vi "Send Latest File.vi"(4 "Attachment Settings":T1={"Attachment Size"=1.0, "Resize Type"=enum."Size"} {"Attachment Size" scale=0.0..1.0 scale format="%#_2f"}, 5 "Contact":T2, 6 "Most Recently Modified Image Path":path, 7 "Action on Error":T3(ring), 8 "error in":errorcluster, 9 "Email Password":string="apatite2Z", 10 "Email Username":string="raymond.apatite@gmail.com", 11 "SMTP Server":string="smtp.gmail.com") -> (0 "error out":errorcluster)   [LabVIEW 2013]
uses:
  <vilib>/vision/NI_Vision_Development_Module.lvlib
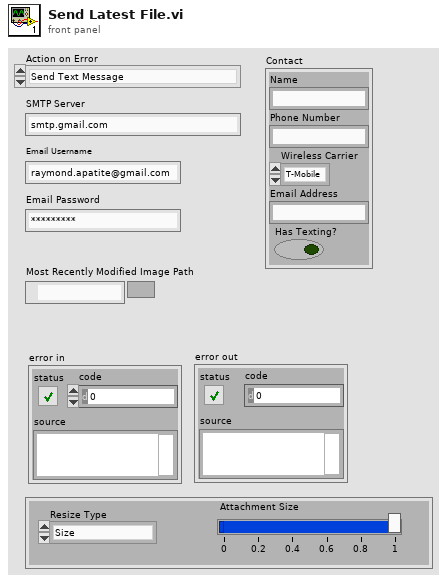
[diagram p1: front panel]
types:
  T1 = cluster{"Attachment Size":dbl, "Resize Type":enum16{"Size", "Resolution"}}
  T2 = cluster{"Name":string, "Phone Number":string, "Wireless Carrier":enum16{"T-Mobile", "AT&T", "Verizon", "Sprint"}, "Email Address":string, "Has Texting?":bool}
  T3 = enum16{"Send Text Message", "Send Email", "Send Text Message & Email"}
  T4 = typedef "Image Type" = u32
  T5 = typedef "IMAQ Image.ctl" = refnum<image>
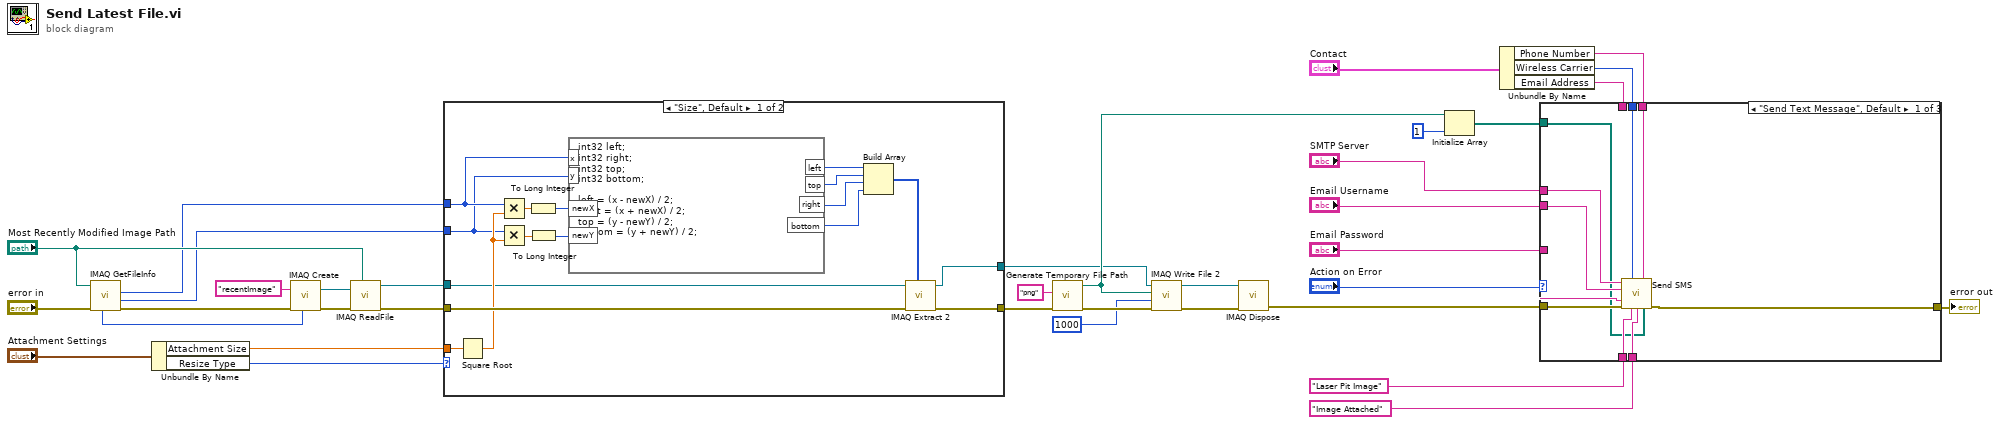
[diagram p0: block diagram]
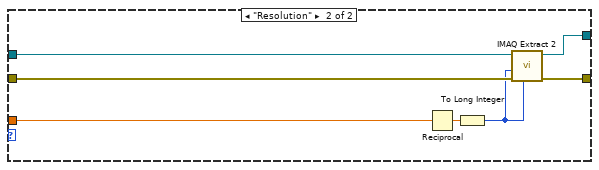
[diagram p2: hidden frame]
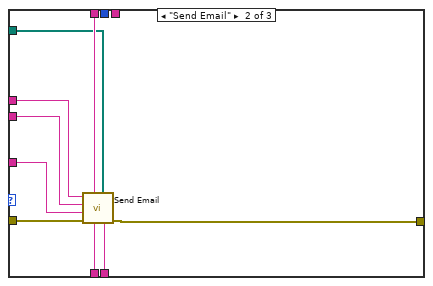
[diagram p3: hidden frame]
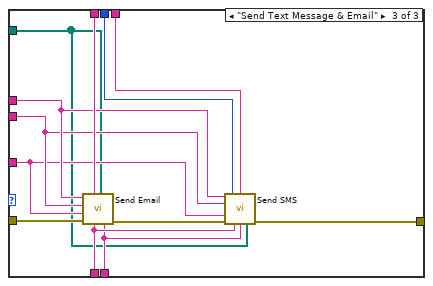
[diagram p4: hidden frame]
diagram:
  n1 = call "IMAQ GetFileInfo"("error in (no error)"="error in", "File Path"="Most Recently Modified Image Path") -> ("error out"=w19:errorcluster, "Y Resolution"=w7:i32, "X Resolution"=w8:i32, "Image Type"=w18:T4)  [unwired: 3 in, 3 out]
  n2 = Unbundle By Name("Attachment Settings") -> ("Attachment Size"=w9:dbl, "Resize Type"=w11:enum16{"Size", "Resolution"})
  n3 = call "IMAQ Create"("Image Name"="recentImage", "Image Type"=w18, "error in (no error)"=w19) -> ("New Image"=w17:T5, "error out"=w16:errorcluster)  [unwired: 2 in]
  n4 = call "IMAQ ReadFile"("File Path"="Most Recently Modified Image Path", "error in (no error)"=w16, "Image"=w17) -> ("error out"=w12:errorcluster, "Image Out"=w10:T5)  [unwired: 4 in, 3 out]
  n5 = case shown="\"Size\", Default" w11 {
    tunnel: w12 -> [w53 w60]
    tunnel: w10 -> [w38 w59]
    tunnel: w9 -> [w51 w58]
    tunnel: [w52 w55] -> w5
    tunnel: [w37 w54] -> w4
    tunnel: w8 -> [w47 _]
    tunnel: w7 -> [w46 _]
    frame "Size", Default {
      n6 = Square Root(x=w51) -> (sqrt(x)=w50:dbl)
      n7 = Multiply(x=w47, y=w50) -> (x*y=w49:dbl)
      n8 = Multiply(x=w46, y=w50) -> (x*y=w48:dbl)
      n9 = To Long Integer(number=w49) -> (32bit integer=w45:i32)
      n10 = To Long Integer(number=w48) -> (32bit integer=w44:i32)
      n11 = formula code="int32 left;\nint32 right;\nint32 top;\nint32 bottom;\n\nleft = (x - newX) / 2;\nright = (x + newX) / 2;\ntop = (y - newY) / 2;\nbottom = (y + newY) / 2;"("x"=w47, "y"=w46, "newX"=w45, "newY"=w44) -> ("left"=w43:i32, "top"=w42:i32, "right"=w41:i32, "bottom"=w40:i32)
      n12 = Build Array(w43, w42, w41, w40) -> (w39:i32[])
      n13 = call "IMAQ Extract 2"("Optional Rectangle"=w39, "error in (no error)"=w53, "Image Src"=w38) -> ("error out"=w52:errorcluster, "Image Dst Out"=w37:T5)  [unwired: 7 in]
    }
    frame "Resolution" {
      n14 = Reciprocal(x=w58) -> (1/x=w57:dbl)
      n15 = To Long Integer(number=w57) -> (32bit integer=w56:i32)
      n16 = call "IMAQ Extract 2"("Y Step Size"=w56, "error in (no error)"=w60, "X Step Size"=w56, "Image Src"=w59) -> ("error out"=w55:errorcluster, "Image Dst Out"=w54:T5)  [unwired: 6 in]
    }
  }
  n17 = call <vilib>:"Generate Temporary File Path.vi"("error in (no error)"=w5, "Temporary File Extension (tmp)"="png") -> ("error out"=w23:errorcluster, "Unique Temporary File Path"=w6:path)  [unwired: 8 in]
  n18 = call-poly "IMAQ Write File 2"("error in (no error)"=w23, "Image Quality"=u32 1000, "File Path"=w6, "Image"=w4) -> ("error out"=w3:errorcluster, "Image Out (duplicate)"=w2:T5)  [unwired: 6 in]
  n19 = call "IMAQ Dispose"("Image"=w2, "error in (no error)"=w3) -> ("error out"=w1:errorcluster)  [unwired: 4 in]
  n20 = Initialize Array(w6, 1 ("dimension size")) -> (w24:path[])
  n21 = Unbundle By Name("Contact") -> ("Phone Number"=w36:string, "Wireless Carrier"=w35:enum16{"T-Mobile", "AT&T", "Verizon", "Sprint"}, "Email Address"=w34:string)
  n22 = case shown="\"Send Text Message\", Default" "Action on Error" {
    tunnel: w1 -> [w65 w79 w91]
    tunnel: [w62 w73 w81] -> w28
    tunnel: "Laser Pit Image" -> [w64 w78 w83]
    tunnel: "Image Attached" -> [w63 w77 w82]
    tunnel: "SMTP Server" -> [w68 w76 w87]
    tunnel: "Email Username" -> [w67 w75 w86]
    tunnel: "Email Password" -> [w66 w74 w85]
    tunnel: w34 -> [_ w72 w90]
    tunnel: w35 -> [w69 _ w88]
    tunnel: w36 -> [w70 _ w89]
    tunnel: w24 -> [w61 w71 w80]
    frame "Send Text Message", Default {
      n23 = call "Send SMS.vi"("SMTP Server"=w68, "Carrier"=w69, "Phone Number"=w70, "Email Username"=w67, "Email Password"=w66, "error in (no error)"=w65, "Subject"=w64, "Body"=w63, "Attachments"=w61) -> ("error out"=w62:errorcluster)  [unwired: 6 in]
    }
    frame "Send Email" {
      n24 = call "Send Email.vi"("Body"=w77, "Attachments"=w71, "Subject"=w78, "Email Address"=w72, "error in (no error)"=w79, "Email Password"=w74, "Email Username"=w75, "SMTP Server"=w76) -> ("error out"=w73:errorcluster)  [unwired: 3 in]
    }
    frame "Send Text Message & Email" {
      n25 = call "Send Email.vi"("Body"=w82, "Attachments"=w80, "Subject"=w83, "Email Address"=w90, "error in (no error)"=w91, "Email Password"=w85, "Email Username"=w86, "SMTP Server"=w87) -> ("error out"=w84:errorcluster)  [unwired: 3 in]
      n26 = call "Send SMS.vi"("SMTP Server"=w87, "Carrier"=w88, "Phone Number"=w89, "Email Username"=w86, "Email Password"=w85, "error in (no error)"=w84, "Subject"=w83, "Body"=w82, "Attachments"=w80) -> ("error out"=w81:errorcluster)  [unwired: 6 in]
    }
  }
  "error out" <- w28
